vi "Read SQLite Connection.vi"(8 "Error In (no error)":errorcluster, 11 "SQLite DB Operator In":refnum<class "SQLite DB Operator.lvclass">) -> (0 "Error Out":errorcluster, 2 "SQLite.lvlib:Connection":refnum<class "Connection.lvclass">, 3 "SQLite DB Operator out":refnum<class "SQLite DB Operator.lvclass">)   [LabVIEW 2023, in "SQLite DB Operator.lvclass"]
uses:
  SQLite DB Operator.lvclass
  <vilib>/drjdpowell/SQLite Library/SQL Connection/Connection.lvclass
  SQLite DB Operator.lvclass/SQLite DB Operator.ctl
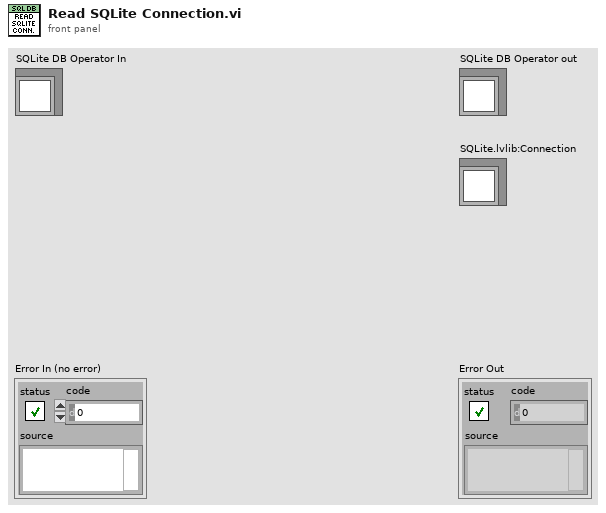
[diagram p1: front panel]
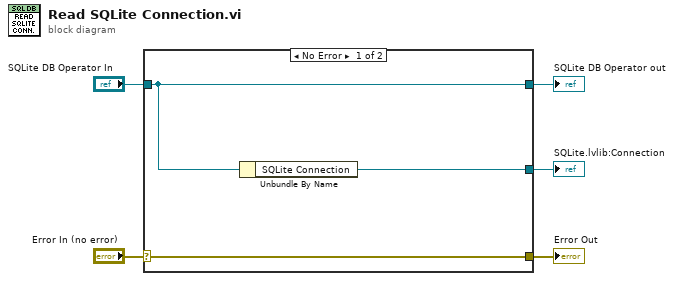
[diagram p0: block diagram]
diagram:
  n1 = case shown="No Error" "Error In (no error)" {
    selector: "Error In (no error)" -> [w8 w9]
    tunnel: [w8 w9] -> w4
    tunnel: [w7 w10] -> w2
    tunnel: "SQLite DB Operator In" -> [w7 w10]
    tunnel: [w6 _] -> w1
    frame No Error {
      n2 = Unbundle By Name(w7) -> ("SQLite Connection"=w6:refnum<class "Connection.lvclass">)
    }
    frame Error {
    }
  }
  "Error Out" <- w4
  "SQLite DB Operator out" <- w2
  "SQLite.lvlib:Connection" <- w1
